vi "testCommandInput.vi"() -> ()   [LabVIEW 2016]
uses:
  dataType.ctl
  CoolerSerialCommand.lvclass
panel:
  in  "Numeric":dbl format="%#_13g"
  out "cmdDataStr":string
  in  "dataType":T1
  out "error out":errorcluster
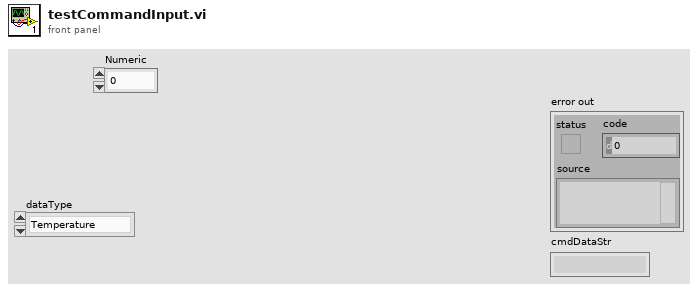
[diagram p1: front panel]
types:
  T1 = typedef "dataType.ctl" = enum16{"Temperature", "Flow", "ControlSensor", "ExternalSensorStatus", "ChillerStatus"}
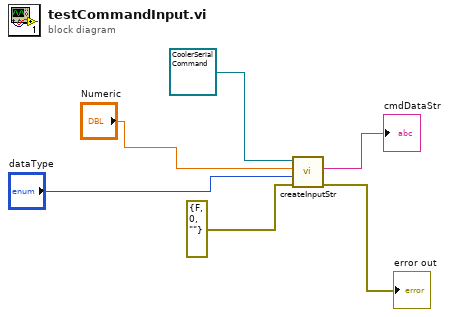
[diagram p0: block diagram]
diagram:
  n1 = call "createInputStr.vi"("error in (no error)"=errorcluster {"status"=FALSE, "code"=0, "source"=""}, "dataType"="dataType", "data"="Numeric", "CoolerSerialCommand in"=refnum<class "CoolerSerialCommand.lvclass"> refnum) -> ("error out"=→"error out":errorcluster, "cmdDataStr"=→"cmdDataStr":string)  [unwired: 5 in, 1 out]
